vi "Validate Item and Invoke Message Creator.vi"(8 "error in (no error)":errorcluster, 11 "Object":T1) -> (0 "error out":errorcluster)   [LabVIEW 2020, in "Message Maker Provider.lvlib"]
uses:
  Message Maker Provider.lvlib
  AFPP Shared/AFPP Shared.lvlib
  <vilib>/ErrorRing/Error Ring.xnode
  AFPP Shared/Validation Mode.ctl
  <vilib>/Utility/error.llb/Error Cluster From Error Code.vi
  <resource>/Framework/Providers/API/ItemRef.ctl
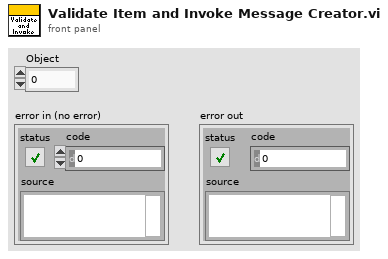
[diagram p1: front panel]
types:
  T1 = typedef "ItemRef.ctl" = u64
  T2 = typedef "AFPP Shared.lvlib/Validation Mode.ctl" = enum16{"An Actor Library", "A Target Tag"}
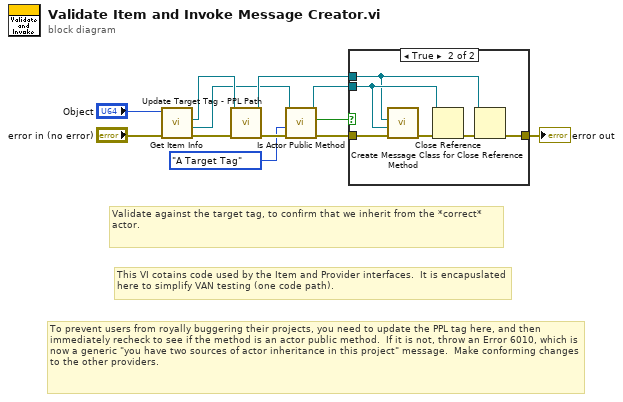
[diagram p0: block diagram]
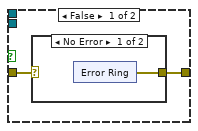
[diagram p2: hidden frame]
diagram:
  # "To prevent users from royally buggering their projects, you need to update the PPL tag here, and then immediately recheck to see if the method is an actor public method.  If it is not, throw an Error 6010, which is now a generic \"you have two sources of actor inheritance in this project\" message.  Make conforming changes to the other providers."
  # "This VI cotains code used by the Item and Provider interfaces.  It is encapuslated here to simplify VAN testing (one code path)."
  # "Validate against the target tag, to confirm that we inherit from the *correct* actor."
  n1 = call "Get Item Info.vi"("error in (no error)"="error in (no error)", "Object"="Object") -> ("error out"=w7:errorcluster, "Item Refnum"=w8:refnum<vi>, "Target"=w10:refnum<vi>)  [unwired: 5 in, 2 out]
  n2 = call "Update Target Tag - PPL Path.vi"("error in (no error)"=w7, "Target"=w10) -> ("error out"=w5:errorcluster, "dup Target"=w11:refnum<vi>)  [unwired: 7 in, 1 out]
  n3 = call "Is Actor Public Method.vi"("error in (no error)"=w5, "Validation"=Validation_Mode."A Target Tag", "ProjectItem in"=w8) -> ("error out"=w6:errorcluster, "Is Actor Public Method"=w12:bool, "ProjectItem out"=w9:refnum<vi>)  [unwired: 5 in, 1 out]
  n4 = case shown="True" w12 {
    tunnel: [w13 w25] -> w3
    tunnel: w6 -> [w14 w24]
    tunnel: w9 -> [_ w23]
    tunnel: w11 -> [_ w22]
    frame False {
      n5 = case shown="No Error" w14 {
        selector: w14 -> [_ w21]
        tunnel: [w15 w21] -> w13
        frame No Error {
          n6 = xnode "Error Ring"() -> ("error out"=w15:errorcluster)
        }
        frame Error {
        }
      }
    }
    frame True {
      n7 = call "Create Message Class for Method.vi"("error in (no error)"=w24, "Item Refnum"=w23, "Target"=w22) -> ("error out"=w27:errorcluster)  [unwired: 6 in, 2 out]
      n8 = Close Reference(reference=w23, error in (no error)=w27) -> (error out=w26:errorcluster)
      n9 = Close Reference(reference=w22, error in (no error)=w26) -> (error out=w25:errorcluster)
    }
  }
  "error out" <- w3
